vi "Gas Chromatograph.vi"() -> ()   [LabVIEW 2012]
uses:
  signal.ctl
  GC record.ctl
  detector.ctl
  zones.ctl
  Tuning.ctl
panel:
  out "updatedisplay":bool
  in  "Min Peak Area":dbl=1.0 min=0.0 format="%.2f"
  in  "tuning":T1={"max noise"=1.0, "min points to fit"=5, "peak threshold"=2.0} {"peak threshold" min=0.0 format="%.2f"; "max noise" min=0.0 format="%.2f"}
  out "zones":T2={"Inj A zone"=TRUE, "Det A zone"=TRUE, "Inj B zone"=TRUE, "Det B zone"=TRUE}
  out "Detectors":T3={"Det A"="FID", "Det B"="TCD"}
  out "Det in use":string
  in  "State":T4
  out "measure sample":bool
  out "method set":bool
  out "data points":u8
  in  "GC record":T5 {"delta x" format="%.2f"; "chromatogram 1" format="%.2f"}
  out "Summary":string[][](table)
  out "delta x":dbl=0.05 format="%.5f"
  out "Signal 1":T6
  out "peaks graph 1":cluster{cluster{"X":dbl, "Y":dbl}[]}[](graph)
  out "chromatogram 1":dbl[](array[numeric]) format="%.2f"
  out "signals":enum16{"signal 1", "signals 1 and 2"}(ring)=enum."signals 1 and 2"
  in  "Serial Port":refnum<visa-resource-name>="COM1"
  out "quit":bool=TRUE
  in  "stop run":bool
  # "time"
  # "area"
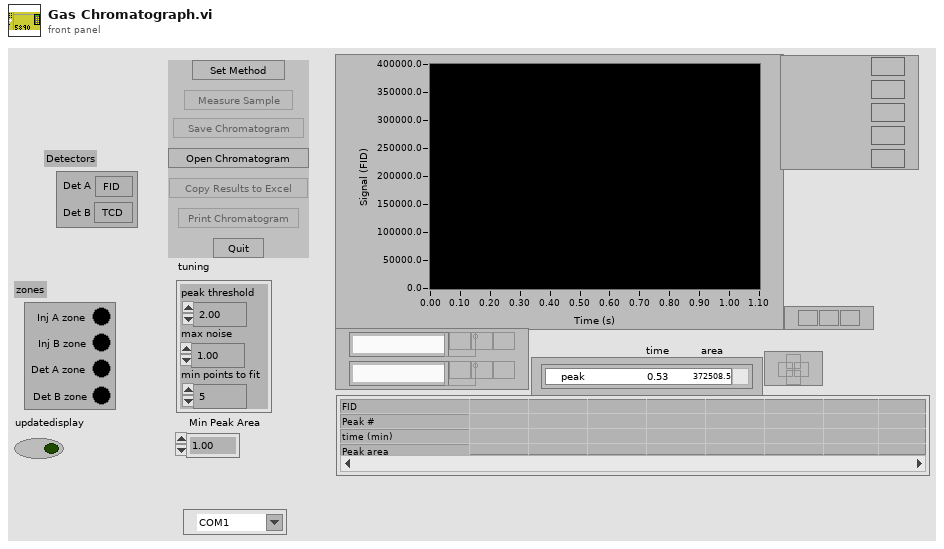
[diagram p1: front panel]
types:
  T1 = typedef "Tuning.ctl" = cluster{"max noise":dbl, "min points to fit":i32, "peak threshold":dbl}
  T2 = typedef "zones.ctl" = cluster{"Inj A zone":bool, "Det A zone":bool, "Inj B zone":bool, "Det B zone":bool}
  T3 = typedef "detector.ctl" = cluster{"Det A":string, "Det B":string}
  T4 = cluster{"Quit":bool, "Set method":bool, "Measure Sample":bool, "Save Chromatogram":bool, "Open Chromatogram":bool, "Copy Results to Excel":bool, "Print Chromatogram":bool}
  T5 = typedef "GC record.ctl" = cluster{"chromatogram 1":dbl[], "Your name":string, "Description":string, "Date":string, "delta x":dbl, "Det in use":string}
  T6 = typedef "signal.ctl" = enum16{"Detector A", "Detector B", "Oven temperature", "Comp 1", "Comp 2", "Inlet A temperature", "Inlet B temperature", "Detector A temperature", "Detector B temperature", "Test Signal"}
  T7 = cluster{"Start X":dbl, "Start Y":dbl, "Summit X":dbl, "Summit Y":dbl, "End X":dbl, "End Y":dbl, "Area":dbl}[]
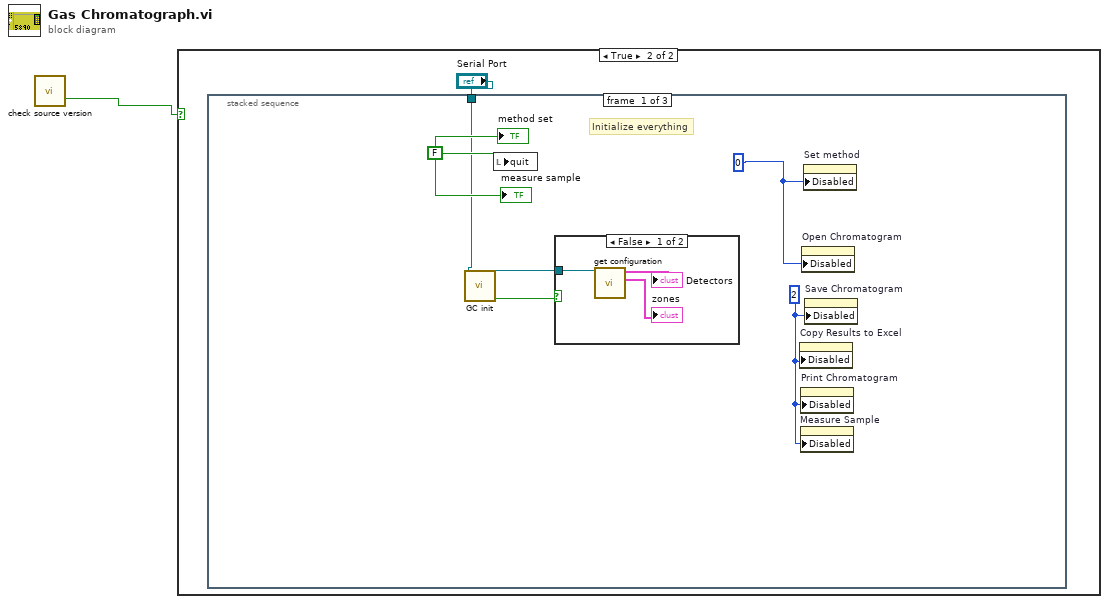
[diagram p0: block diagram]
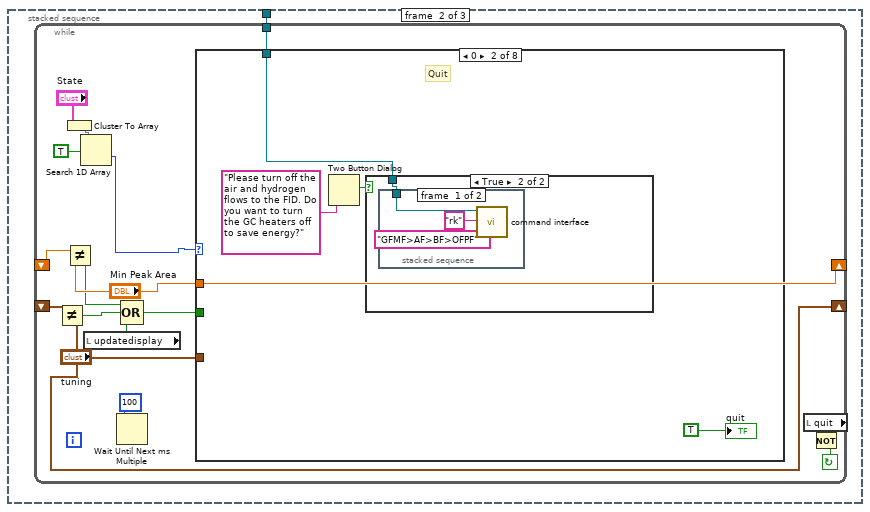
[diagram p4: hidden frame]
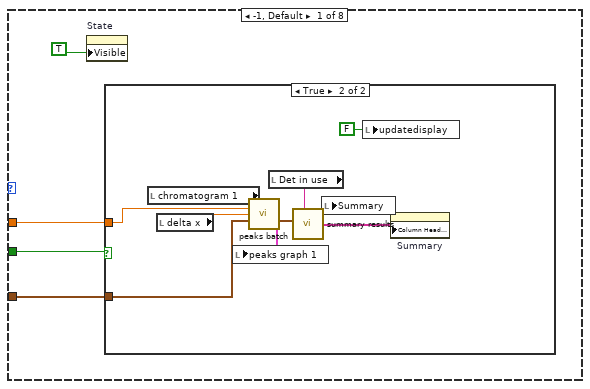
[diagram p5: hidden frame]
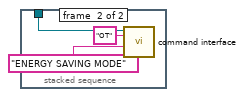
[diagram p8: hidden frame]
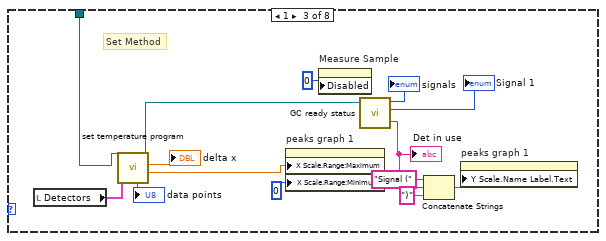
[diagram p9: hidden frame]
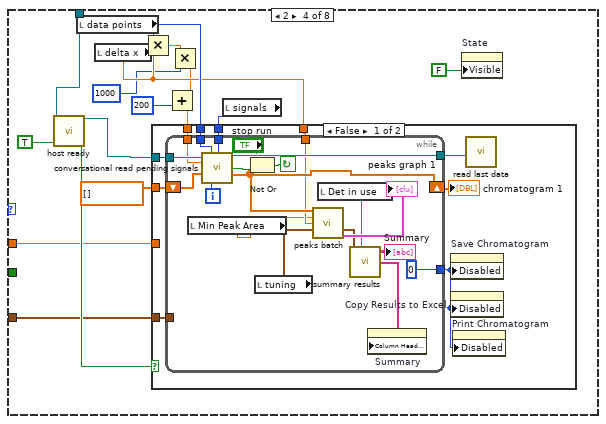
[diagram p10: hidden frame]
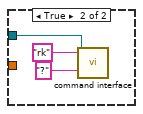
[diagram p11: hidden frame]
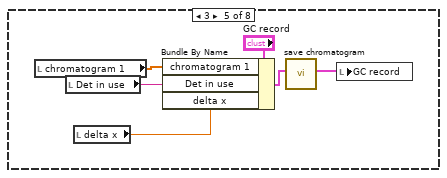
[diagram p12: hidden frame]
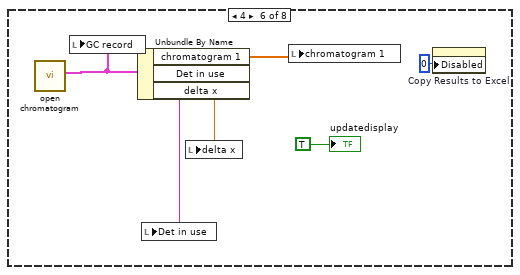
[diagram p13: hidden frame]
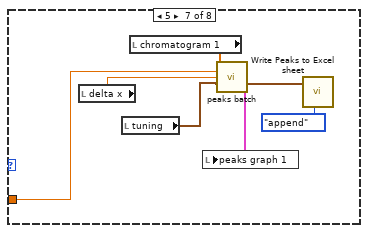
[diagram p14: hidden frame]
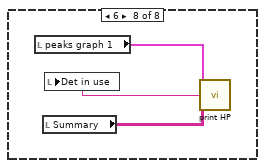
[diagram p15: hidden frame]
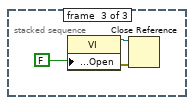
[diagram p16: hidden frame]
diagram:
  n1 = call "check source version.vi"() -> ("continue running?"=w1:bool)  [unwired: 2 in, 3 out]
  n2 = case shown="True" w1 {
    frame False {
    }
    frame True {
      n3 = stacked-sequence {
        tunnel: "Serial Port" -> [w7 w12 _]
        frame #0 {
          w4 = 2
          w3 = 0
          w8 = FALSE
          # "Initialize everything"
          n4 = call "GC init.vi"("Serial Port"=w7) -> ("error"=w5:bool, "Serial Port"=w6:refnum<visa-resource-name>)  [unwired: 9 in]
          n5 = local write "quit"(w8) -> ()
          n6 = case shown="False" w5 {
            tunnel: w6 -> [w11 _]
            frame False {
              n7 = call "get configuration.vi"("Serial Port"=w11) -> ("zones"=→"zones":T2, "Detectors"=→"Detectors":T3)  [unwired: 5 in, 1 out]
            }
            frame True {
            }
          }
          n8 = property on="Copy Results to Excel" class="Bool"("Disabled"=w4) -> ()  [unwired: 2 in, 2 out]
          n9 = property on="Print Chromatogram" class="Bool"("Disabled"=w4) -> ()  [unwired: 2 in, 2 out]
          n10 = property on="Measure Sample" class="Bool"("Disabled"=w4) -> ()  [unwired: 2 in, 2 out]
          n11 = property on="Open Chromatogram" class="Bool"("Disabled"=w3) -> ()  [unwired: 2 in, 2 out]
          n12 = property on="Set method" class="Bool"("Disabled"=w3) -> ()  [unwired: 2 in, 2 out]
          n13 = property on="Save Chromatogram" class="Bool"("Disabled"=w4) -> ()  [unwired: 2 in, 2 out]
          "method set" <- w8
          "measure sample" <- w8
        }
        frame #1 {
          n14 = while {
            shift-left: _ -> [w17]
            shift-right: ["Min Peak Area"] -> _
            shift-left: _ -> [w19]
            shift-right: ["tuning"] -> _
            tunnel: w12 -> [w26]
            stop <- w28 continue-if-true
            n15 = Not Equal?(x=w19, y="tuning") -> (x != y?=w15:bool)
            n16 = Cluster To Array(cluster="State") -> (array=w24:bool[])
            n17 = Not Equal?(x=w17, y="Min Peak Area") -> (x != y?=w16:bool)
            n18 = Search 1D Array(1D array=w24, element=TRUE) -> (index of element=w21:i32)  [unwired: 1 in]
            n19 = local read "updatedisplay"() -> (w13:bool)
            n20 = Wait Until Next ms Multiple(millisecond multiple=100) -> ()  [unwired: 1 out]
            n21 = Compound Arithmetic op=OR(w16, w15, w13) -> (w14:bool)
            n22 = case shown="0" w21 {
              tunnel: w26 -> [_ w43 w66 w80 _ _ _ _]
              tunnel: w14 -> [w32 _ _ _ _ _ _ _]
              tunnel: "tuning" -> [w30 _ _ w69 _ _ _ _]
              tunnel: "Min Peak Area" -> [w29 _ _ w68 _ _ w129 _]
              frame -1, Default {
                n23 = property on="State" class="Clust"("Visible"=TRUE) -> ()  [unwired: 2 in, 2 out]
                n24 = case shown="True" w32 {
                  tunnel: w30 -> [_ w35]
                  tunnel: w29 -> [_ w34]
                  frame False {
                  }
                  frame True {
                    n25 = local read "chromatogram 1"() -> (w41:dbl[])
                    n26 = local read "delta x"() -> (w42:dbl)
                    n27 = call "peaks batch.vi"("signal in"=w41, "Min Peak Area"=w34, "X Interval"=w42, "tuning parameters"=w35) -> ("Peaks"=w36:T7, "graph data"=w40:cluster{cluster{"X":dbl, "Y":dbl}[]}[])  [unwired: 9 in, 1 out]
                    n28 = local write "peaks graph 1"(w40) -> ()
                    n29 = local read "Det in use"() -> (w37:string)
                    n30 = call "summary results.vi"("Det in use"=w37, "Peaks"=w36) -> ("summary"=w38:string[][], 7:w39:string[])  [unwired: 4 in, 1 out]
                    n31 = local write "Summary"(w38) -> ()
                    n32 = local write "updatedisplay"(FALSE ("updatedisplay")) -> ()
                    n33 = property on="Summary" class="Tbl (strict)"("Column Header Strings[]"=w39) -> ()  [unwired: 2 in, 2 out]
                  }
                }
              }
              frame 0 {
                # "Quit"
                n34 = Two Button Dialog(message="Please turn off the air and hydrogen flows to the FID. Do you want to turn the GC heaters off to save energy?") -> (T button?=w45:bool)  [unwired: 2 in]
                n35 = case shown="True" w45 {
                  tunnel: w43 -> [_ w47]
                  frame False {
                  }
                  frame True {
                    n36 = stacked-sequence {
                      tunnel: w47 -> [w50 w51]
                      frame #0 {
                        n37 = call "command interface.vi"("Parameter"="GFMF>AF>BF>OFPF", "command"="rk", "Serial Port"=w50) -> ()  [unwired: 4 in, 4 out]
                      }
                      frame #1 {
                        n38 = call "command interface.vi"("Parameter"="ENERGY SAVING MODE", "command"="OT", "Serial Port"=w51) -> ()  [unwired: 4 in, 4 out]
                      }
                    }
                  }
                }
                "quit" <- TRUE
              }
              frame 1 {
                # "Set Method"
                n39 = local read "Detectors"() -> (w60:T3)
                n40 = call "set temperature program.vi"("Detectors"=w60, "Serial Port"=w66) -> ("run time"=w65:dbl, "delta x"=→"delta x":dbl, "Serial Port"=w63:refnum<visa-resource-name>, "data points"=→"data points":u8)  [unwired: 5 in, 1 out]
                n41 = property on="peaks graph 1" class="XYGraph (strict)"("X Scale.Range:Maximum"=w65, "X Scale.Range:Minimum"=0) -> ()  [unwired: 2 in, 2 out]
                n42 = property on="Measure Sample" class="Bool"("Disabled"=0) -> ()  [unwired: 2 in, 2 out]
                n43 = call "GC ready status.vi"("Serial Port"=w63) -> ("signals"=→"signals":enum16{"signal 1", "signals 1 and 2"}, "Signal 1"=→"Signal 1":T6, "Det in use"=w56:string)  [unwired: 4 in, 3 out]
                "Det in use" <- w56
                n44 = Concatenate Strings("Signal (" ("Substring"), w56, ")" ("Substring")) -> (w57:string)
                n45 = property on="peaks graph 1" class="XYGraph (strict)"("Y Scale.Name Label.Text"=w57) -> ()  [unwired: 2 in, 2 out]
              }
              frame 2 {
                n46 = call "host ready.vi"("Serial Port"=w80, "start run"=TRUE) -> ("Serial Port"=w82:refnum<visa-resource-name>, "canceled"=w79:bool)  [unwired: 10 in, 2 out]
                n47 = local read "data points"() -> (w77:u8)
                n48 = local read "delta x"() -> (w76:dbl)
                n49 = Multiply(x=w77, y=w76) -> (x*y=w75:dbl)
                n50 = Multiply(x=w75, y=1000) -> (x*y=w71:dbl)
                n51 = Add(x=w71, y=200) -> (x+y=w73:dbl)
                n52 = local read "signals"() -> (w83:enum16{"signal 1", "signals 1 and 2"})
                n53 = case shown="False" w79 {
                  tunnel: w82 -> [w93 w114]
                  tunnel: dbl[] [] ("Output Array") -> [w91 _]
                  tunnel: w83 -> [w88 _]
                  tunnel: w77 -> [w87 _]
                  tunnel: w76 -> [w86 _]
                  tunnel: w73 -> [w85 _]
                  tunnel: w69 -> [w84 _]
                  tunnel: w68 -> [_ _]
                  frame False {
                    n54 = while {
                      tunnel: w84 -> [_]
                      tunnel: w85 -> [w103]
                      tunnel: w86 -> [w101]
                      tunnel: w87 -> [w105]
                      tunnel: w88 -> [w106]
                      tunnel: [w107] -> w89
                      tunnel: [0] -> w90
                      shift-left: w91 -> [w111]
                      shift-right: [w102] -> w92
                      tunnel: w93 -> [w108]
                      i -> [w109]
                      stop <- w113 continue-if-true
                      n55 = local read "Min Peak Area"() -> (w95:dbl)
                      n56 = call "conversational read pending signals.vi"("Serial Port"=w108, "data points"=w105, "signals"=w106, "Max time (ms)"=w103, "signal 1 in"=w111, "i"=w109) -> ("Serial Port"=w107:refnum<visa-resource-name>, "run done"=w110:bool, "signal 1 out"=w102:dbl[])  [unwired: 5 in, 2 out]
                      n57 = Not Or(1:w110, 2:"stop run") -> (0:w113:bool)
                      n58 = local read "tuning"() -> (w94:T1)
                      n59 = call "peaks batch.vi"("signal in"=w102, "Min Peak Area"=w95, "X Interval"=w101, "tuning parameters"=w94) -> ("Peaks"=w99:T7, "graph data"=→"peaks graph 1":cluster{cluster{"X":dbl, "Y":dbl}[]}[])  [unwired: 9 in, 1 out]
                      n60 = local read "Det in use"() -> (w96:string)
                      n61 = call "summary results.vi"("Det in use"=w96, "Peaks"=w99) -> ("summary"=→"Summary":string[][], 7:w97:string[])  [unwired: 4 in, 1 out]
                      n62 = property on="Summary" class="Tbl (strict)"("Column Header Strings[]"=w97) -> ()  [unwired: 2 in, 2 out]
                    }
                    "chromatogram 1" <- w92
                    n63 = property on="Save Chromatogram" class="Bool"("Disabled"=w90) -> ()  [unwired: 2 in, 2 out]
                    n64 = property on="Copy Results to Excel" class="Bool"("Disabled"=w90) -> ()  [unwired: 2 in, 2 out]
                    n65 = property on="Print Chromatogram" class="Bool"("Disabled"=w90) -> ()  [unwired: 2 in, 2 out]
                    n66 = call "read last data.vi"("Serial Port"=w89) -> ()  [unwired: 9 in, 2 out]
                  }
                  frame True {
                    n67 = call "command interface.vi"("Parameter"="?", "command"="rk", "Serial Port"=w114) -> ()  [unwired: 4 in, 4 out]
                  }
                }
                n68 = property on="State" class="Clust"("Visible"=FALSE) -> ()  [unwired: 2 in, 2 out]
              }
              frame 3 {
                n69 = local read "chromatogram 1"() -> (w121:dbl[])
                n70 = local read "Det in use"() -> (w117:string)
                n71 = local read "delta x"() -> (w120:dbl)
                n72 = Bundle By Name(cluster="GC record", "chromatogram 1"=w121, "Det in use"=w117, "delta x"=w120) -> (w122:T5)
                n73 = call "save chromatogram.vi"("GC record"=w122) -> ("GC record"=w119:T5)  [unwired: 6 in]
                n74 = local write "GC record"(w119) -> ()
              }
              frame 4 {
                n75 = call "open chromatogram.vi"() -> ("GC record"=w128:T5)  [unwired: 7 in]
                n76 = local write "GC record"(w128) -> ()
                n77 = Unbundle By Name(w128) -> ("chromatogram 1"=w124:dbl[], "Det in use"=w127:string, "delta x"=w125:dbl)
                n78 = local write "Det in use"(w127) -> ()
                n79 = local write "delta x"(w125) -> ()
                n80 = local write "chromatogram 1"(w124) -> ()
                n81 = property on="Copy Results to Excel" class="Bool"("Disabled"=u8 0) -> ()  [unwired: 2 in, 2 out]
                "updatedisplay" <- TRUE ("updatedisplay")
              }
              frame 5 {
                n82 = local read "delta x"() -> (w135:dbl)
                n83 = local read "tuning"() -> (w133:T1)
                n84 = local read "chromatogram 1"() -> (w134:dbl[])
                n85 = call "peaks batch.vi"("signal in"=w134, "Min Peak Area"=w129, "X Interval"=w135, "tuning parameters"=w133) -> ("Peaks"=w130:T7, "graph data"=w132:cluster{cluster{"X":dbl, "Y":dbl}[]}[])  [unwired: 9 in, 1 out]
                n86 = local write "peaks graph 1"(w132) -> ()
                n87 = call "Write Peaks to Excel sheet.vi"("action"=enum16{"open", "append", "close"}."append", "Peaks"=w130) -> ()  [unwired: 9 in, 1 out]
              }
              frame 6 {
                n88 = local read "peaks graph 1"() -> (w138:cluster{cluster{"X":dbl, "Y":dbl}[]}[])
                n89 = local read "Summary"() -> (w136:string[][])
                n90 = call "print HP.vi"("peaks graph 1"=w138, "table in"=w136) -> ("Det in use"=w137:string)  [unwired: 13 in]
                n91 = local write "Det in use"(w137) -> ()
              }
            }
            n92 = local read "quit"() -> (w27:bool)
            n93 = Not(x=w27) -> (.not. x?=w28:bool)
          }
        }
        frame #2 {
          n94 = property class="VI"("Front Panel Window:Open"=FALSE) -> (reference out=w139:refnum<vi>, error out=w140:errorcluster)  [unwired: 2 in]
          n95 = Close Reference(reference=w139, error in (no error)=w140) -> ()  [unwired: 1 out]
        }
      }
    }
  }
